vi "Set SCFG wrapper.vi"(0 "dwDevIndex":u32, 5 "dwCanNodeId":u32, 9 "SCFG_INFO_OBJ In":T1, 11 "error in (no error)":errorcluster caption="错误输入（无错误）") -> (4 "function return":u32, 10 "SCFG_INFO_OBJ Out":T1, 15 "error out":errorcluster caption="错误输出")   [LabVIEW 2016, in "UISimCanFunc_wrapper.lvlib"]
doc: "_declspec (dllexport) DWORD SetSCFG_wrapper(DWORD dwDevIndex, DWORD dwCanNodeId, P_S12CON pS12CON, P_S34CON pS34CON,\n P_DUMMY_SCFG_INFO_OBJ pDummySCFGInfo);"
uses:
  <userlib>/UISimCanFunc_wrapper/UISimCanFunc_wrapper.lvlib
  <userlib>/UISimCanFunc_wrapper/ctl/SCFG_INFO_OBJ.ctl
  <userlib>/UISimCanFunc_wrapper/ctl/S12CON.ctl
  <userlib>/UISimCanFunc_wrapper/ctl/S34CON.ctl
  <userlib>/UISimCanFunc_wrapper/UISimCanFunc_wrapper.dll
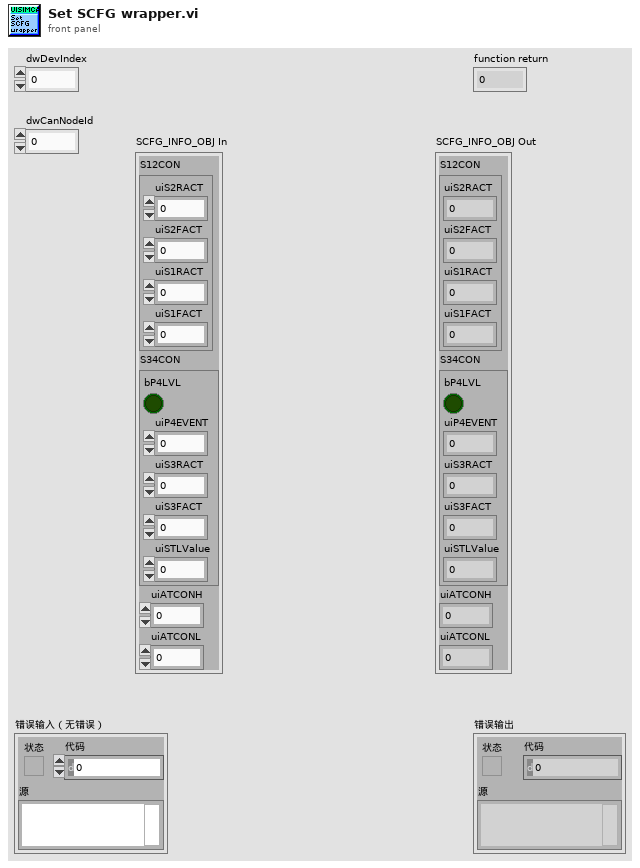
[diagram p1: front panel]
types:
  T1 = typedef "UISimCanFunc_wrapper.lvlib/SCFG_INFO_OBJ.ctl" = cluster{"S12CON":T2, "S34CON":T3, "uiATCONH":u32, "uiATCONL":u32}
  T2 = typedef "UISimCanFunc_wrapper.lvlib/S12CON.ctl" = cluster{"uiS2RACT":u32, "uiS2FACT":u32, "uiS1RACT":u32, "uiS1FACT":u32}
  T3 = typedef "UISimCanFunc_wrapper.lvlib/S34CON.ctl" = cluster{"bP4LVL":bool, "uiP4EVENT":u32, "uiS3RACT":u32, "uiS3FACT":u32, "uiSTLValue":u32}
  T4 = cluster{"bP4LVL":i32, "uiP4EVENT":u32, "uiS3RACT":u32, "uiS3FACT":u32, "uiSTLValue":u32}
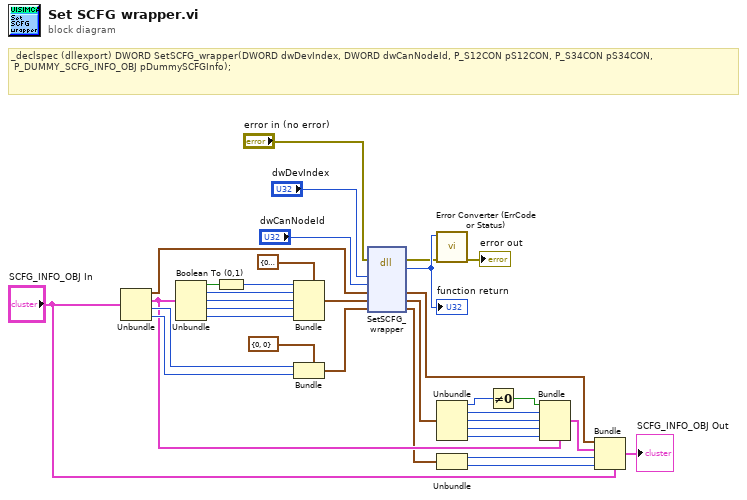
[diagram p0: block diagram]
diagram:
  # "_declspec (dllexport) DWORD SetSCFG_wrapper(DWORD dwDevIndex, DWORD dwCanNodeId, P_S12CON pS12CON, P_S34CON pS34CON,\n\tP_DUMMY_SCFG_INFO_OBJ pDummySCFGInfo);"
  n1 = Unbundle("SCFG_INFO_OBJ In") -> ("S12CON"=w28:T2, "S34CON"=w10:T3, "uiATCONH"=w26:u32, "uiATCONL"=w25:u32)
  n2 = Unbundle(w10) -> ("bP4LVL"=w17:bool, "uiP4EVENT"=w21:u32, "uiS3RACT"=w20:u32, "uiS3FACT"=w19:u32, "uiSTLValue"=w18:u32)
  n3 = Boolean To (0,1)(Boolean=w17) -> (0, 1=w16:i16)
  n4 = Bundle(cluster=T4 {"bP4LVL"=0, "uiP4EVENT"=0, "uiS3RACT"=0, "uiS3FACT"=0, "uiSTLValue"=0} ("pS34CON out"), "bP4LVL"=w16, "uiP4EVENT"=w21, "uiS3RACT"=w20, "uiS3FACT"=w19, "uiSTLValue"=w18) -> (w22:T4)
  n5 = Bundle(cluster=cluster{"uiATCONH":u32, "uiATCONL":u32} {"uiATCONH"=0, "uiATCONL"=0} ("pDummySCFGInfo"), "uiATCONH"=w26, "uiATCONL"=w25) -> (w24:cluster{"uiATCONH":u32, "uiATCONL":u32})
  n6 = dll-call lib="C:/Program Files (x86)/National Instruments/LabVIEW 2016/user.lib/UISimCanFunc_wrapper/UISimCanFunc_wrapper.*" fn="SetSCFG_wrapper"(error in="error in (no error)", "dwDevIndex"="dwDevIndex", "dwCanNodeId"="dwCanNodeId", "pS12CON"=w28, "pS34CON"=w22, "pDummySCFGInfo"=w24) -> (error out=w30:errorcluster, w34:u32, "pS12CON"=w13:T2, "pS34CON"=w12:T4, "pDummySCFGInfo"=w3:cluster{"uiATCONH":u32, "uiATCONL":u32})  [unwired: 4 in, 1 out]
  "function return" <- w34
  n7 = call <userlib>:"Error Converter (ErrCode or Status).vi"("error in (no error)"=w30, "error code"=w34) -> ("error out"=→"error out":errorcluster)  [unwired: 9 in]
  n8 = Unbundle(w12) -> ("bP4LVL"=w11:i32, "uiP4EVENT"=w8:u32, "uiS3RACT"=w7:u32, "uiS3FACT"=w6:u32, "uiSTLValue"=w5:u32)
  n9 = Unbundle(w3) -> ("uiATCONH"=w2:u32, "uiATCONL"=w1:u32)
  n10 = Not Equal To 0?(x=w11) -> (x != 0?=w9:bool)
  n11 = Bundle(cluster=w10, "bP4LVL"=w9, "uiP4EVENT"=w8, "uiS3RACT"=w7, "uiS3FACT"=w6, "uiSTLValue"=w5) -> (w4:T3)
  n12 = Bundle(cluster="SCFG_INFO_OBJ In", "S12CON"=w13, "S34CON"=w4, "uiATCONH"=w2, "uiATCONL"=w1) -> (→"SCFG_INFO_OBJ Out":T1)
